vi "Serial_format.vi"(0 "Serial in":refnum<class "Serial.lvclass">, 5 "bits":dbl=8.0, 7 "parity":T1(ring), 9 "stop bits":dbl=1.0, 11 "error in (no error)":errorcluster) -> (4 "Serial out":refnum<class "Serial.lvclass">, 15 "error out":errorcluster)   [LabVIEW 2011, in "mbed_LVLibrary.lvlib" / "Serial.lvclass"]
uses:
  Serial.lvclass
  Serial.lvclass/Serial.ctl
  Transport Mechanisms/mbed/mbed.lvclass
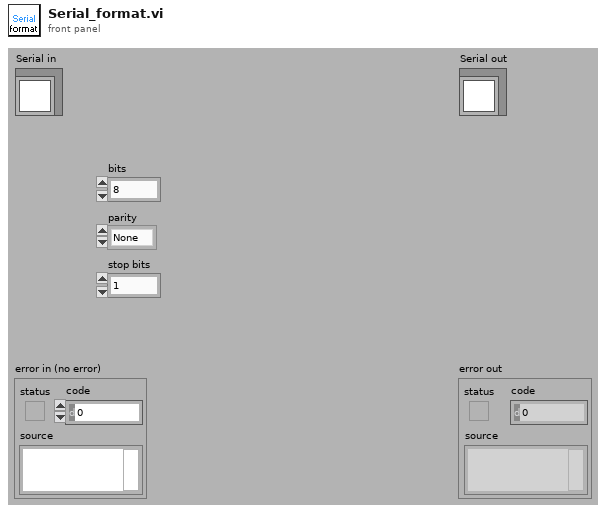
[diagram p1: front panel]
types:
  T1 = enum16{"None", "Odd", "Even", "Forced1", "Forced0"}
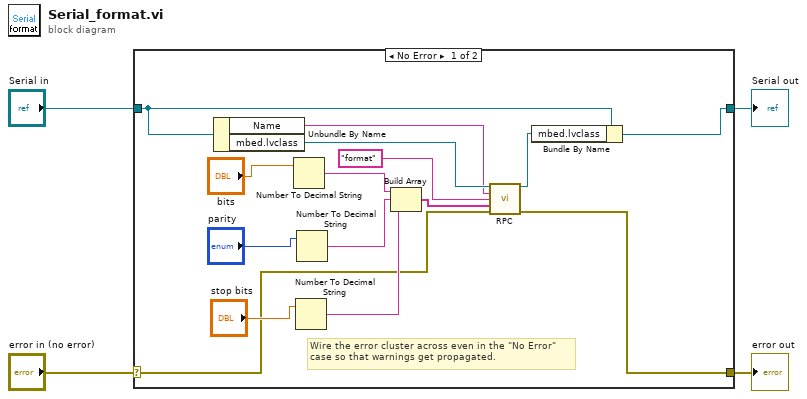
[diagram p0: block diagram]
diagram:
  n1 = case shown="No Error" "error in (no error)" {
    selector: "error in (no error)" -> [w6 w21]
    tunnel: [w5 w21] -> w3
    tunnel: [w7 w20] -> w1
    tunnel: "Serial in" -> [w8 w20]
    frame No Error {
      # "Wire the error cluster across even in the \"No Error\"\ncase so that warnings get propagated."
      n2 = Unbundle By Name(w8) -> ("Name"=w12:string, "mbed.lvclass"=w13:refnum<class "mbed.lvclass">)
      n3 = Number To Decimal String(number="bits") -> (decimal integer string=w16:string)  [unwired: 1 in]
      n4 = Number To Decimal String(number="stop bits") -> (decimal integer string=w14:string)  [unwired: 1 in]
      n5 = Number To Decimal String(number="parity") -> (decimal integer string=w15:string)  [unwired: 1 in]
      n6 = Build Array(w16, w15, w14) -> (w10:string[])
      n7 = call-dynamic "RPC.vi"("mbed in"=w13, "Name"=w12, "method"="format", "Args"=w10, "error in (no error)"=w6) -> ("mbed out"=w9:refnum<class "mbed.lvclass">, "error out"=w5:errorcluster)  [unwired: 8 in, 1 out]
      n8 = Bundle By Name(cluster=w8, "mbed.lvclass"=w9) -> (w7:refnum<class "Serial.lvclass">)
    }
    frame Error {
    }
  }
  "error out" <- w3
  "Serial out" <- w1
